vi "WristGetBeforeClampSetpoint.vi"() -> (3 "WristGetBeforeClampSetpoint":dbl)   [LabVIEW 2023]
uses:
  WristGlobal.vi
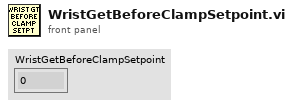
[diagram p1: front panel]
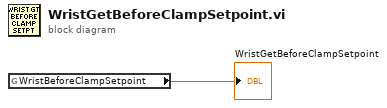
[diagram p0: block diagram]
diagram:
  n1 = global read "WristGlobal.vi" "WristBeforeClampSetpoint"() -> (→"WristGetBeforeClampSetpoint":dbl)
